vi "Global 1.vi"() -> ()   [LabVIEW 2020]
panel:
  in  "String":string=" "
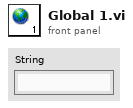
[diagram p1: front panel]
diagram:
